vi "Wiper Internal.vi"(9 "Close?":bool, 10 "MotorControlDevRef":T1={"DeviceStatus"={"status"=FALSE, "code"=0, "source"=""}, "Type"=enum."PWM", "PWM"={"Controller"=enum."Controller 1", "PWM Channel"=enum."Invalid", "DeadBand"={"Name"="", "maxPositivePwm"=0, "minPositivePwm"=0, "centerPwm"=0, "maxNegativePwm"=0, "minNegativePwm"=0, "angularRange"=0}}, "CAN"={"Device Number"=0, "Control Mode"=enum."Percent VBus", "Semaphore"=refnum, "Max Vout"=12.0, "TalonSRX Control Mode"=enum."Percent VBus"}, "Invert"=FALSE, "TransformRef"=refnum, "InvTransformRef"=refnum}) -> (2 "Done?":bool)   [LabVIEW 2014]
doc: "Opens/closes the can grabber by running a loop until either a limit switch switches or the current changes dramatically."
uses:
  <vilib>/Rock Robotics/WPI/MotorControl/WPI_MotorControlDeviceRef.ctl
  <vilib>/Rock Robotics/WPI/MotorControl/WPI_MotorControlType.ctl
  <vilib>/Rock Robotics/SystemInterfaces/Typedef/FPGA_TypedefDigitalModule.ctl
  <vilib>/Rock Robotics/SystemInterfaces/DIO/FPGA_DIOPWMChannel.ctl
  <vilib>/Rock Robotics/WPI/PWM/WPI_PWMDeadband.ctl
  <vilib>/Rock Robotics/WPI/CAN/Jaguar/SubVIs/WPI_CANJaguar_ControlMode.ctl
  <vilib>/Rock Robotics/WPI/CAN/TalonSRX/WPI_CANTalonSRX_APIControlMode.ctl
  <vilib>/Rock Robotics/WPI/PWM/WPI_PWMTransform_ConPane.ctl
  Robot Global Data.vi
panel:
  in  "Holding Power":dbl=0.2 format="%#_13g"
  in  "Closing Speed":dbl=1.0 format="%#_13g"
  in  "Opening Speed":dbl=-1.0 format="%#_13g"
  # "Positive Closes\nNegative Opens"
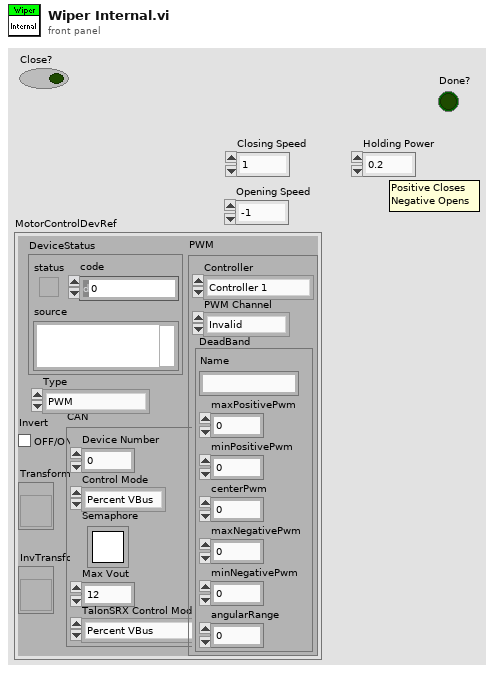
[diagram p1: front panel]
types:
  T1 = typedef "WPI_MotorControlDeviceRef.ctl" = cluster{"DeviceStatus":errorcluster, "Type":T2, "PWM":cluster{"Controller":T3, "PWM Channel":T4, "DeadBand":T5}, "CAN":cluster{"Device Number":u8, "Control Mode":T6, "Semaphore":T7, "Max Vout":dbl, "TalonSRX Control Mode":T8}, "Invert":bool, "TransformRef":T9, "InvTransformRef":T9}
  T2 = typedef "WPI_MotorControlType.ctl" = enum16{"PWM", "CAN", "CANTalonSRX"}
  T3 = typedef "FPGA_TypedefDigitalModule.ctl" = enum16{"Controller 1"}
  T4 = typedef "FPGA_DIOPWMChannel.ctl" = enum8{"PWM 0", "PWM 1", "PWM 2", "PWM 3", "PWM 4", "PWM 5", "PWM 6", "PWM 7", "PWM 8", "PWM 9", "PWM MXP 0", "PWM MXP 1", "PWM MXP 2", "PWM MXP 3", "PWM MXP 4", "PWM MXP 5", "PWM MXP 6", "PWM MXP 7", "PWM MXP 8", "PWM MXP 9", "Invalid"}
  T5 = typedef "WPI_PWMDeadband.ctl" = cluster{"Name":string, "maxPositivePwm":i32, "minPositivePwm":i32, "centerPwm":i32, "maxNegativePwm":i32, "minNegativePwm":i32, "angularRange":u16}
  T6 = typedef "WPI_CANJaguar_ControlMode.ctl" = enum8{"Percent VBus", "Current", "Speed", "Position", "Voltage"}
  T7 = typedef "Semaphore RefNum" = refnum<k1>
  T8 = typedef "WPI_CANTalonSRX_APIControlMode.ctl" = enum8{"Percent VBus", "Speed", "Position", "Slave", "Unchanged / Invalid"}
  T9 = typedef "WPI_PWMTransform_ConPane.ctl" = refnum<vi>
  T10 = typedef "WPI_CANTalonSRX_GlobalStatus.ctl" = cluster{"Applied Throttle":dbl, "Module Enabled":bool, "CAN Error":errorcluster, "Closed Loop Error":dbl, "Forward Limit Switch Closed":bool, "Reverse Limit Switch Closed":bool, "Sensor Position":dbl, "Sensor Velocity":dbl, "Current":dbl, "Sticky Fault - Over Temp":bool, "Sticky Fault - Under Voltage":bool, "Sticky Fault - Forward Limit":bool, "Sticky Fault - Reverse Limit":bool, "Sticky Fault - Forward Soft Limit":bool, "Sticky Fault - Reverse Soft Limit":bool, "Brake is Enabled":bool, "Encoder Position":dbl, "Encoder Velocity":dbl, "Encoder Index Count":dbl, "Encoder A Pin State":bool, "Encoder B Pin State":bool, "Encoder Index Pin State":bool, "Analog In":dbl, "Analog In Velocity":dbl, "Temperature (C)":dbl, "Battery Voltage":dbl}
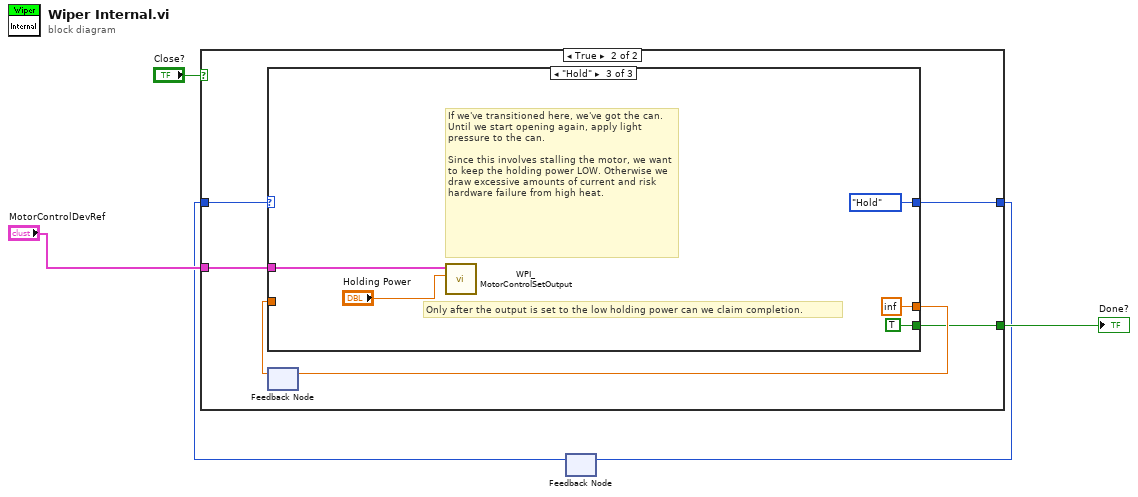
[diagram p0: block diagram]
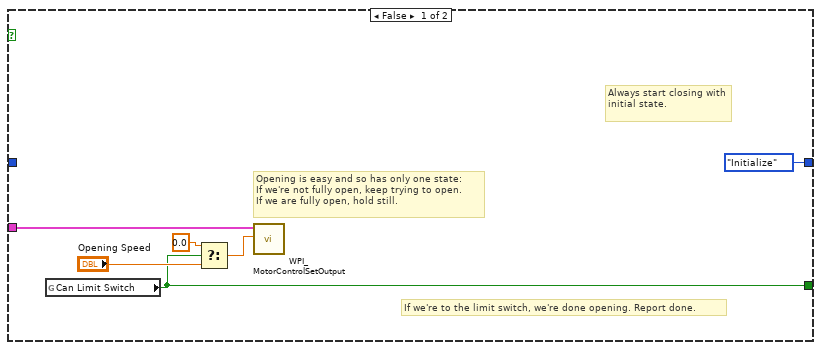
[diagram p2: hidden frame]
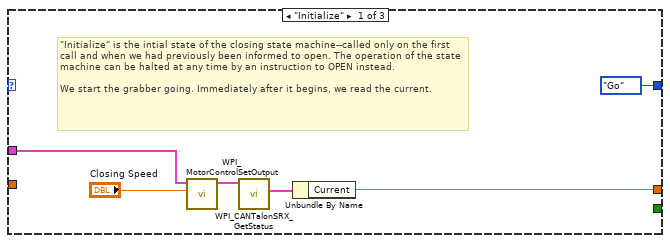
[diagram p3: hidden frame]
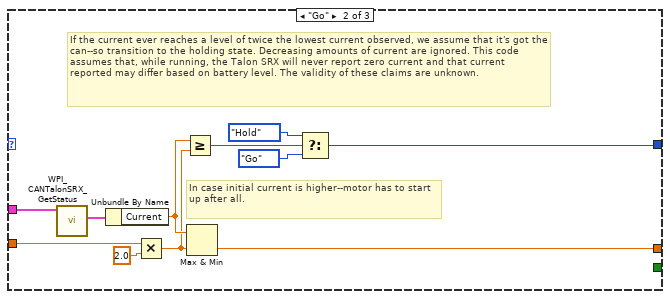
[diagram p4: hidden frame]
diagram:
  n1 = feedback #1() -> (w1:enum16{"Initialize", "Go", "Hold"})  [unwired: 1 in]
  n2 = case shown="True" "Close?" {
    tunnel: "MotorControlDevRef" -> [w11 w17]
    tunnel: w1 -> [_ w16]
    tunnel: [enum16{"Initialize", "Go", "Hold"}."Initialize" w13] -> w2
    tunnel: [w6 w12] -> w4
    frame False {
      # "Always start closing with initial state."
      # "If we're to the limit switch, we're done opening. Report done."
      # "Opening is easy and so has only one state:\nIf we're not fully open, keep trying to open.\nIf we are fully open, hold still."
      n3 = global read "Robot Global Data.vi" "Can Limit Switch"() -> (w6:bool)
      n4 = Select(t=0.0, s=w6, f="Opening Speed") -> (s? t:f=w10:dbl)
      n5 = call <vilib>:"WPI_MotorControlSetOutput.vi"("Output"=w10, "MotorControlDevRef"=w11) -> ()  [unwired: 7 in, 3 out]
    }
    frame True {
      n6 = feedback #2() -> (w14:dbl)  [unwired: 1 in]
      n7 = case shown="\"Hold\"" w16 {
        tunnel: w17 -> [w23 w33 w35]
        tunnel: [w19 w28 inf ("Current")] -> w15
        tunnel: w14 -> [_ w31 _]
        tunnel: [enum16{"Initialize", "Go", "Hold"}."Go" w24 enum16{"Initialize", "Go", "Hold"}."Hold"] -> w13
        tunnel: [_ _ TRUE] -> w12
        frame "Initialize" {
          # "\"Initialize\" is the intial state of the closing state machine--called only on the first call and when we had previously been informed to open. The operation of the state machine can be halted at any time by an instruction to OPEN instead.\n \nWe start the grabber going. Immediately after it begins, we read the current."
          n8 = call <vilib>:"WPI_MotorControlSetOutput.vi"("Output"="Closing Speed", "MotorControlDevRef"=w23) -> ("MotorControlDevRef"=w20:T1)  [unwired: 7 in, 2 out]
          n9 = call <vilib>:"WPI_CANTalonSRX_GetStatus.vi"("CAN Talon SRX Ref"=w20) -> ("Talon SRX Status"=w22:T10)  [unwired: 8 in, 2 out]
          n10 = Unbundle By Name(w22) -> ("Current"=w19:dbl)
        }
        frame "Go" {
          # "If the current ever reaches a level of twice the lowest current observed, we assume that it's got the can--so transition to the holding state. Decreasing amounts of current are ignored. This code assumes that, while running, the Talon SRX will never report zero current and that current reported may differ based on battery level. The validity of these claims are unknown."
          # "In case initial current is higher--motor has to start up after all."
          n11 = call <vilib>:"WPI_CANTalonSRX_GetStatus.vi"("CAN Talon SRX Ref"=w33) -> ("Talon SRX Status"=w34:T10)  [unwired: 8 in, 2 out]
          n12 = Unbundle By Name(w34) -> ("Current"=w30:dbl)
          n13 = Multiply(x=w31, y=2.0) -> (x*y=w29:dbl)
          n14 = Greater Or Equal?(x=w30, y=w29) -> (x >= y?=w25:bool)
          n15 = Max & Min(x=w30, y=w29) -> (min(x,y)=w28:dbl)  [unwired: 1 out]
          n16 = Select(t=enum16{"Initialize", "Go", "Hold"}."Hold", s=w25, f=enum16{"Initialize", "Go", "Hold"}."Go") -> (s? t:f=w24:enum16{"Initialize", "Go", "Hold"})
        }
        frame "Hold" {
          # "Only after the output is set to the low holding power can we claim completion."
          # "If we've transitioned here, we've got the can. Until we start opening again, apply light pressure to the can.\n\nSince this involves stalling the motor, we want to keep the holding power LOW. Otherwise we draw excessive amounts of current and risk hardware failure from high heat."
          n17 = call <vilib>:"WPI_MotorControlSetOutput.vi"("Output"="Holding Power", "MotorControlDevRef"=w35) -> ()  [unwired: 7 in, 3 out]
        }
      }
      n18 = feedback-in #2(w15) -> ()
    }
  }
  "Done?" <- w4
  n19 = feedback-in #1(w2) -> ()
